vi "Low Pass Filter.vi"(10 "LP Frequency":dbl, 11 "Audio Data":dbl[](array[numeric])) -> (3 "Low Pass Audio Data":dbl[](array[numeric]))   [LabVIEW 2018, in "Channel.lvclass"]
uses:
  Channel.lvclass
  <vilib>/Analysis/3filter.llb/Filter Passband Type.ctl
  Libraries/Globals/Constants.vi
  <vilib>/Analysis/3filter.llb/Bessel Filter (DBL).vi
  <vilib>/Analysis/NI_AALBase.lvlib
  Libraries/Globals/Globals.lvlib
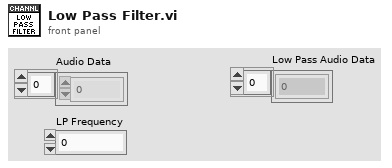
[diagram p1: front panel]
types:
  T1 = typedef "NI_AALBase.lvlib/Filter Passband Type.ctl" = enum32{"Lowpass", "Highpass", "Bandpass", "Bandstop"}
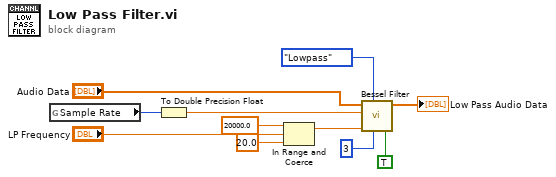
[diagram p0: block diagram]
diagram:
  n1 = global read "Constants.vi" "Sample Rate"() -> (w4:i32)
  n2 = To Double Precision Float(number=w4) -> (double precision float=w3:dbl)
  n3 = In Range and Coerce(upper limit=20000.0 ("y"), x="LP Frequency", lower limit=20.0) -> (coerced(x)=w7:dbl)  [unwired: 1 out]
  n4 = call-poly <vilib>:"Bessel Filter.vi"("init/cont (init:F)"=TRUE, "order"=3, "filter type"=Filter_Passband_Type."Lowpass", "low cutoff freq: fl"=w7, "sampling freq: fs"=w3, "X"="Audio Data") -> ("Filtered X"=→"Low Pass Audio Data":dbl[])  [unwired: 2 in, 1 out]
